vi "Label to Index.vi"(8 "error in (no error)":errorcluster, 10 "Label":string, 11 "VacuumLines in":refnum<class "VacuumLines.lvclass">) -> (0 "error out":errorcluster, 2 "Index":i32, 3 "VacuumLines out":refnum<class "VacuumLines.lvclass">)   [LabVIEW 2016, in "Hardware.lvlib" / "VacuumLine.lvlib" / "VacuumLines.lvclass"]
uses:
  <userlib>/Common Components/Hardware/Abstract System/VacuumLine/VacuumLines/VacuumLines.lvclass
  <userlib>/Common Components/Hardware/Abstract System/VacuumLine/VacuumLines/VacuumLines.lvclass/VacuumLines.ctl
  <userlib>/Common Components/Hardware/Abstract System/VacuumLine/VacuumLine/VacuumLine.lvclass/VacuumLine.ctl
  <userlib>/Common Components/Hardware/Abstract System/VacuumLine/VacuumLine/Read Label.vi
  <userlib>/Common Components/Hardware/Abstract System/VacuumLine/VacuumLine/VacuumLine.lvclass
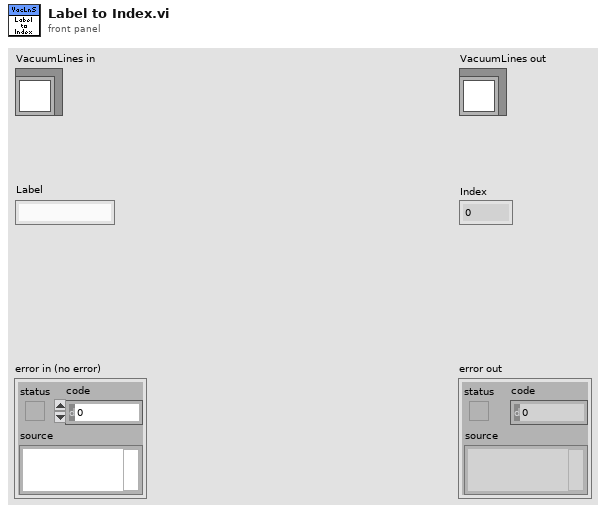
[diagram p1: front panel]
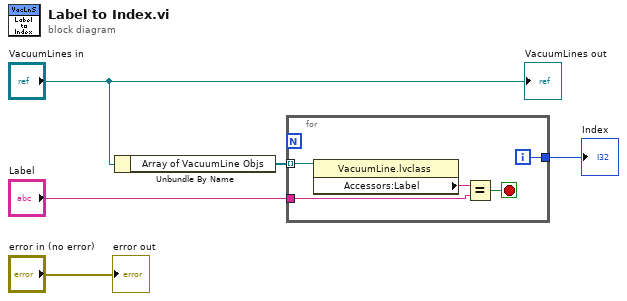
[diagram p0: block diagram]
diagram:
  n1 = Unbundle By Name("VacuumLines in") -> ("Array of VacuumLine Objs"=w3:refnum<class "VacuumLine.lvclass">[])
  n2 = for {
    tunnel: w3 -> [w10] mode=indexing
    tunnel: "Label" -> [w8]
    tunnel: [w6] -> w1
    i -> [w6]
    stop <- w7 stop-if-true
    n3 = property class="VacuumLine.lvclass"(reference=w10) -> ("Accessors:Label"=w9:string)  [unwired: 1 in, 2 out]
    n4 = Equal?(x=w9, y=w8) -> (x = y?=w7:bool)
  }
  "Index" <- w1
  "error out" <- "error in (no error)"
  "VacuumLines out" <- "VacuumLines in"
